vi "Get Objects Available for PDO Mapping.vi"(8 "Error In":errorcluster, 10 "Type":enum16{"TX PDO", "RX PDO"}(ring), 11 "reference in":refnum<class "Electronic Datasheet.lvclass">) -> (0 "Error Out":errorcluster, 2 "Objects Available for PDO Mapping":refnum<class "OD Entry.lvclass">[](array[class]), 3 "reference out":refnum<class "Electronic Datasheet.lvclass">)   [LabVIEW 2024, in "Electronic Datasheet.lvlib" / "Electronic Datasheet.lvclass"]
uses:
  Electronic Datasheet.lvclass
  Core/OD Entry/OD Entry.lvclass
  Electronic Datasheet.lvclass/Electronic Datasheet.ctl
  Core/Sorted Object Dictionary/Sorted Object Dictionary.lvclass
  Core/PDO Mapping Type.ctl
  Core/Electronic Datasheet.lvlib
  Core/Object Type.ctl
  Core/OD Sub-Entry/OD Sub-Entry.lvclass
  D:/git/EDS-File-Viewer/source/Core/OD Entry/OD Entry.lvclass
  D:/git/EDS-File-Viewer/source/Core/OD Sub-Entry/OD Sub-Entry.lvclass
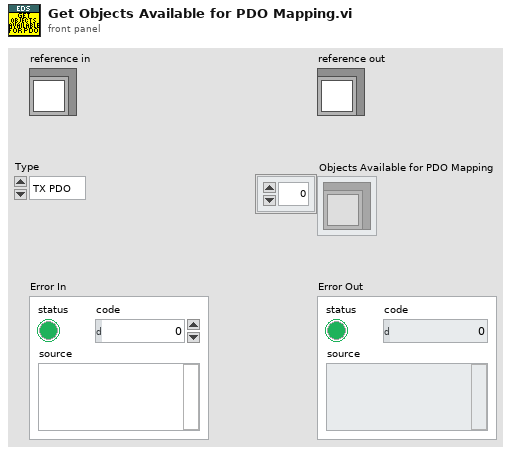
[diagram p1: front panel]
types:
  T1 = typedef "Electronic Datasheet.lvlib/PDO Mapping Type.ctl" = enum16{"no", "optional", "RPDO", "TPDO", "UNKNOWN"}
  T2 = typedef "Electronic Datasheet.lvlib/Electronic Datasheet.lvclass/ObjectAttributes.ctl" = cluster{"EDS File Path":path, "Object Dict":refnum<class "Dictionary.lvclass">, "Sorted Object Dict":refnum<class "Sorted Object Dictionary.lvclass">, "Device Info":refnum<class "Device Info.lvclass">, "File Info":refnum<class "File Info.lvclass">}
  T3 = typedef "Electronic Datasheet.lvlib/Object Type.ctl" = u8
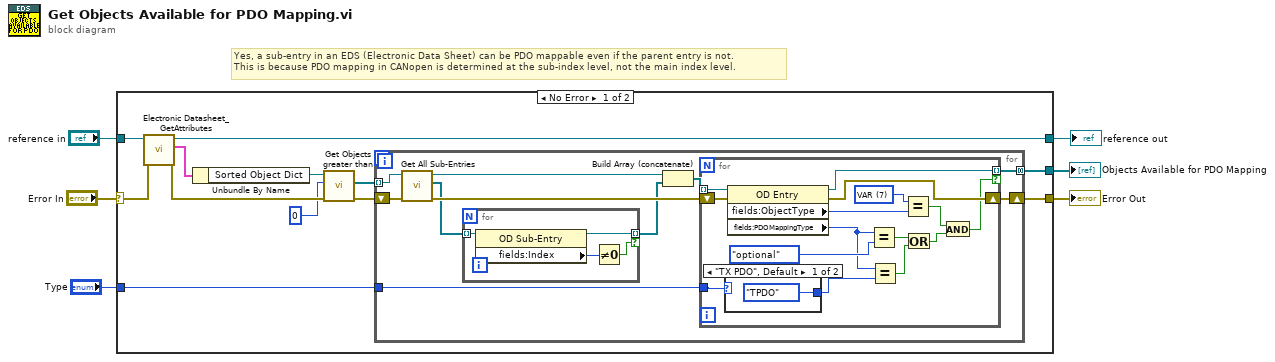
[diagram p0: block diagram]
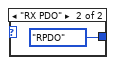
[diagram p2: hidden frame]
diagram:
  # "Yes, a sub-entry in an EDS (Electronic Data Sheet) can be PDO mappable even if the parent entry is not.\nThis is because PDO mapping in CANopen is determined at the sub-index level, not the main index level."
  n1 = case shown="No Error" "Error In" {
    selector: "Error In" -> [w18 w51]
    tunnel: [w8 w51] -> w5
    tunnel: [w15 w50] -> w3
    tunnel: "reference in" -> [w16 w50]
    tunnel: "Type" -> [w10 _]
    tunnel: [w9 _] -> w1
    frame No Error {
      n2 = call "Electronic Datasheet_GetAttributes.vi"("Error In"=w18, "reference in"=w16) -> ("Error Out"=w13:errorcluster, "Data"=w17:T2, "reference out"=w15:refnum<class "Electronic Datasheet.lvclass">)  [unwired: 6 in, 1 out]
      n3 = Unbundle By Name(w17) -> ("Sorted Object Dict"=w14:refnum<class "Sorted Object Dictionary.lvclass">)
      n4 = call "Get Objects greater than.vi"("error in"=w13, "Lower Bound"=u16 0, "Sorted Object Dictionary in"=w14) -> ("error out"=w11:errorcluster, "Entries"=w12:refnum<class "OD Entry.lvclass">[])  [unwired: 6 in, 1 out]
      n5 = for {
        tunnel: w12 -> [w25] mode=indexing
        tunnel: w10 -> [w27]
        tunnel: [w23] -> w9 mode=concatenating
        shift-right: [w26] -> w8
        shift-left: w11 -> [w28]
        n6 = call "Get All Sub-Entries.vi"("Error In"=w28, "reference in"=w25) -> ("Error Out"=w24:errorcluster, "Sub-Entries"=w21:refnum<class "OD Sub-Entry.lvclass">[], "reference out"=w22:refnum<class "OD Entry.lvclass">)  [unwired: 6 in, 1 out]
        n7 = for {
          tunnel: w21 -> [w49] mode=indexing
          tunnel: [w48] -> w20 mode=indexing if=w47
          n8 = property class="OD Sub-Entry"(reference=w49) -> (reference out=w48:refnum<class "OD Sub-Entry.lvclass">, "fields:Index"=w46:u16)  [unwired: 1 in, 1 out]
          n9 = Not Equal To 0?(x=w46) -> (x != 0?=w47:bool)
        }
        n10 = Build Array (concatenate)(w22, w20) -> (w19:refnum<class "OD Entry.lvclass">[])
        n11 = for {
          tunnel: w27 -> [w43]
          tunnel: [w40] -> w23 mode=indexing if=w29
          tunnel: w19 -> [w30] mode=indexing
          shift-right: [w42] -> w26
          shift-left: w24 -> [w41]
          w37 = T3 7 items=["NULL"=0, "DOMAIN"=2, "DEFTYPE"=5, "DEFSTRUCT"=6, "VAR"=7, "ARRAY"=8, "RECORD"=9] ("y")
          n12 = case shown="\"TX PDO\", Default" w43 {
            tunnel: [PDO_Mapping_Type."TPDO" ("y") PDO_Mapping_Type."RPDO" ("y")] -> w33
            frame "TX PDO", Default {
            }
            frame "RX PDO" {
            }
          }
          n13 = property class="OD Entry"(reference=w30, error in=w41) -> (reference out=w40:refnum<class "OD Entry.lvclass">, error out=w42:errorcluster, "fields:ObjectType"=w38:T3, "fields:PDOMappingType"=w34:T1)
          n14 = Equal?(x=w34, y=PDO_Mapping_Type."optional") -> (x = y?=w36:bool)
          n15 = Equal?(x=w34, y=w33) -> (x = y?=w35:bool)
          n16 = Equal?(x=w37, y=w38) -> (x = y?=w31:bool)
          n17 = Or(x=w36, y=w35) -> (x .or. y?=w32:bool)
          n18 = And(x=w31, y=w32) -> (x .and. y?=w29:bool)
        }
      }
    }
    frame Error {
    }
  }
  "Error Out" <- w5
  "reference out" <- w3
  "Objects Available for PDO Mapping" <- w1
